vi "Find Register Offset.vi"(8 "error in (no error)":errorcluster, 10 "register name":string, 11 "session in":u32) -> (0 "error out":errorcluster, 2 "resource offset":u32, 3 "session out":u32)   [LabVIEW 2020, in "FPGA Register IO.lvlib"]
uses:
  FPGA Register IO.lvlib
  TypeDefs/Register Data Store.ctl
  NiFpga.dll
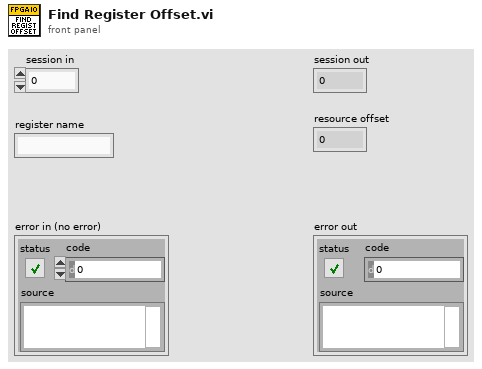
[diagram p1: front panel]
types:
  T1 = typedef "FPGA Register IO.lvlib/Register Data Store.ctl" = cluster{"Register Names":string[], "Register Offset":u32[]}
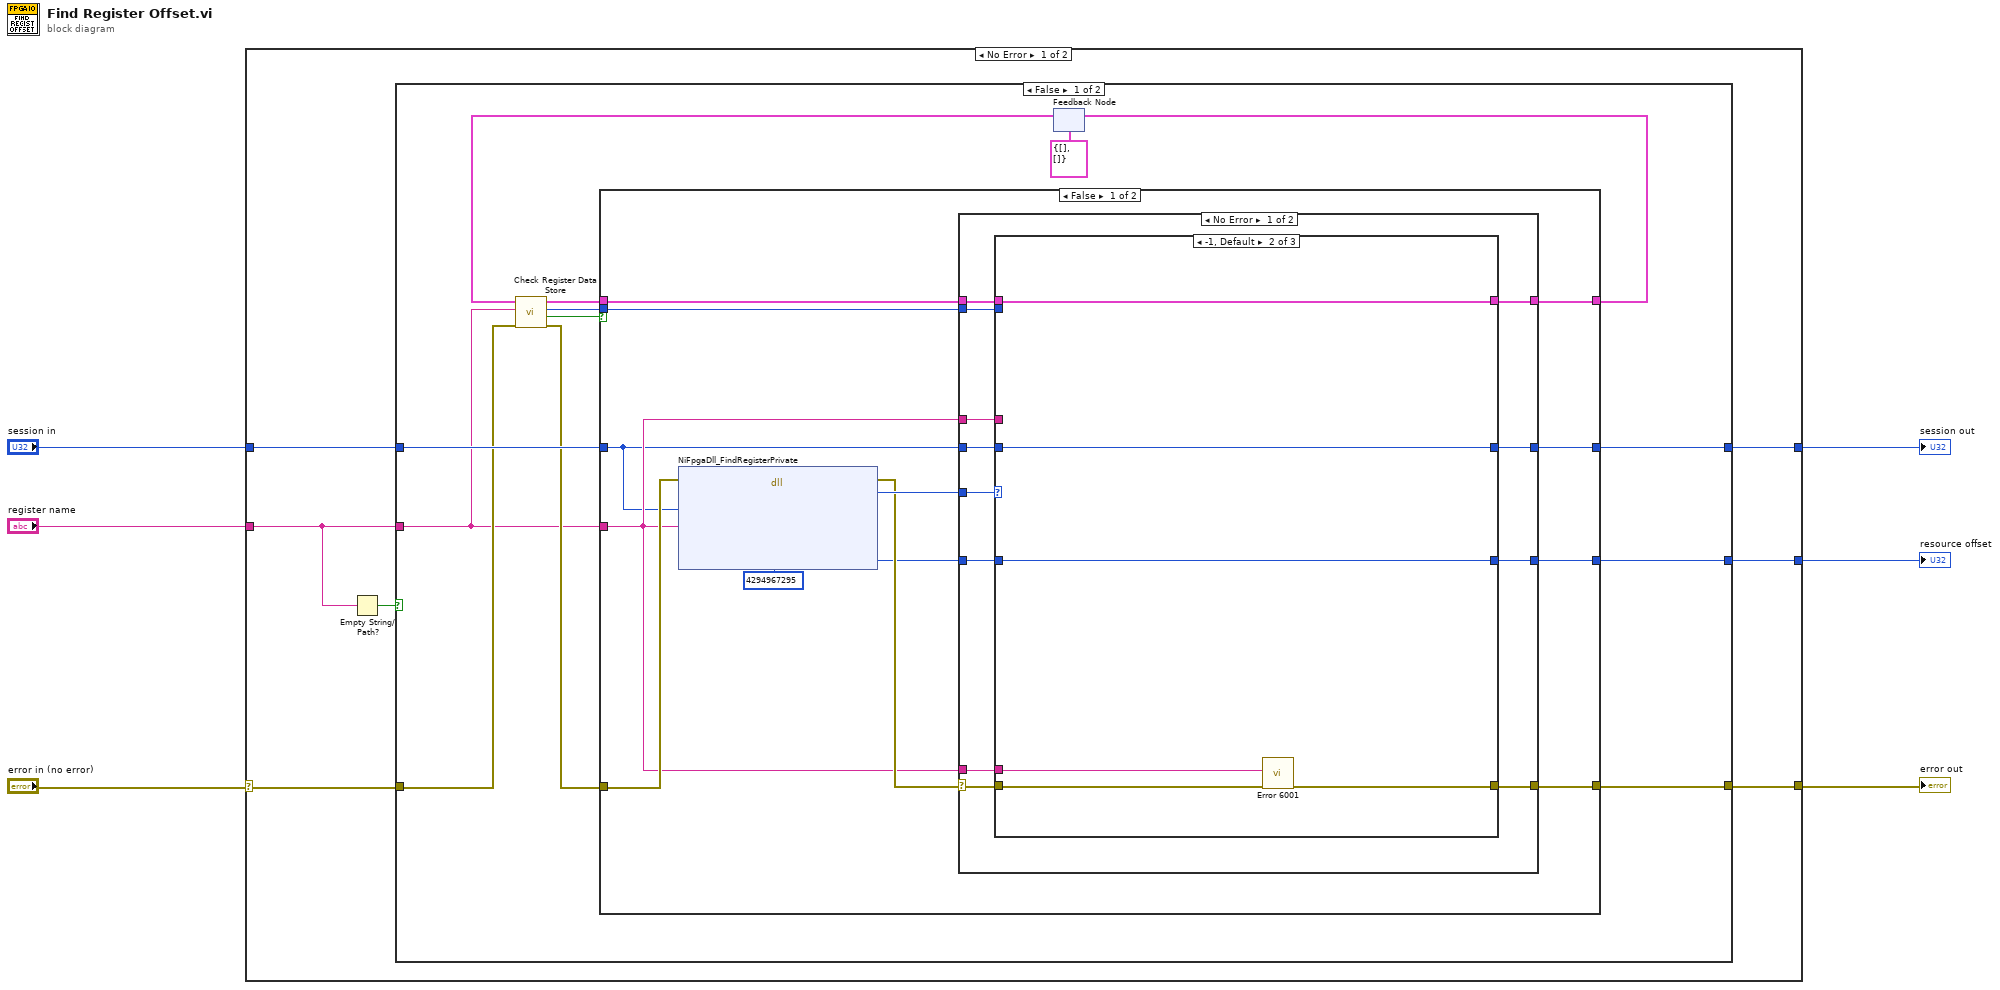
[diagram p0: block diagram]
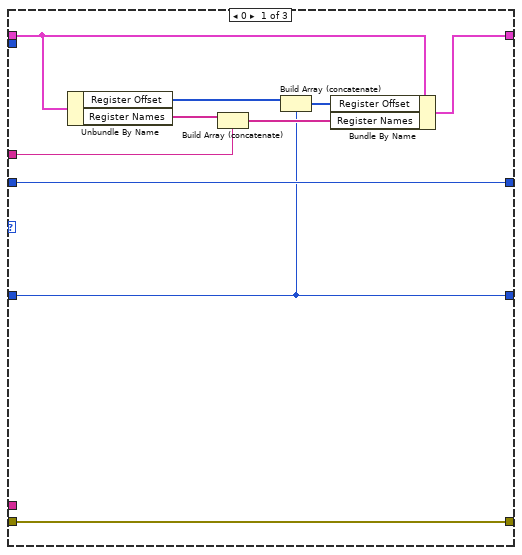
[diagram p2: hidden frame]
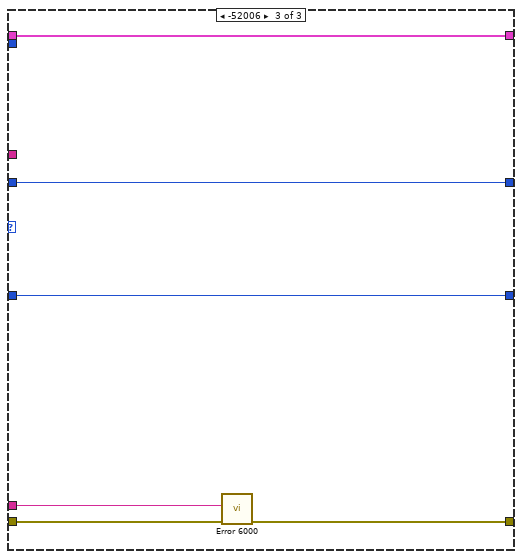
[diagram p3: hidden frame]
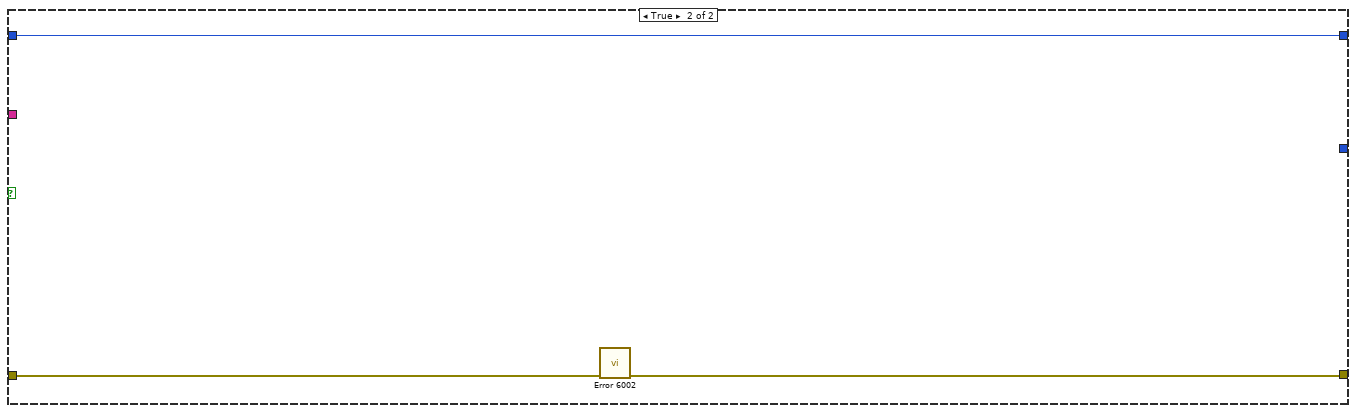
[diagram p6: hidden frame]
diagram:
  n1 = case shown="No Error" "error in (no error)" {
    selector: "error in (no error)" -> [w9 w86]
    tunnel: [w12 w86] -> w3
    tunnel: "register name" -> [w8 _]
    tunnel: "session in" -> [w13 w85]
    tunnel: [w11 w85] -> w4
    tunnel: [w10 _] -> w2
    frame No Error {
      n2 = Empty String/Path?(string/path=w8) -> (empty?=w7:bool)
      n3 = case shown="False" w7 {
        tunnel: w13 -> [w26 w82]
        tunnel: [w25 w83] -> w12
        tunnel: [w24 w82] -> w11
        tunnel: [w23 _] -> w10
        tunnel: w9 -> [w17 w84]
        tunnel: w8 -> [w14 _]
        frame False {
          n4 = feedback #1(T1 {"Register Names"=[], "Register Offset"=[]}) -> (w21:T1)
          n5 = call "Check Register Data Store.vi"("error in (no error)"=w17, "register name"=w14, "register data store in"=w21) -> ("error IO"=w16:errorcluster, "Found"=w15:bool, "register offset"=w19:u32, "register data store out"=w20:T1)  [unwired: 5 in]
          n6 = case shown="False" w15 {
            tunnel: w16 -> [w38 w80]
            tunnel: w26 -> [w29 w81]
            tunnel: [w27 w78] -> w23
            tunnel: [w36 w80] -> w25
            tunnel: [w28 w81] -> w24
            tunnel: w14 -> [w32 _]
            tunnel: w20 -> [w34 w79]
            tunnel: w19 -> [w33 w78]
            tunnel: [w30 w79] -> w18
            frame False {
              n7 = dll-call lib="NiFpga.*" fn="NiFpgaDll_FindRegisterPrivate"(error in=w38, "session"=w29, "registerName"=w32, "expectedResourceType"=u32 4294967295) -> (error out=w35:errorcluster, "status"=w37:i32, "resourceOffset"=w31:u32)  [unwired: 6 in, 1 out]
              n8 = case shown="No Error" w35 {
                selector: w35 -> [w48 w77]
                tunnel: w37 -> [w51 _]
                tunnel: [w50 w77] -> w36
                tunnel: w32 -> [w49 _]
                tunnel: w34 -> [w47 w74]
                tunnel: w33 -> [w46 _]
                tunnel: w32 -> [w45 _]
                tunnel: w31 -> [w44 w75]
                tunnel: [w43 w74] -> w30
                tunnel: w29 -> [w42 w76]
                tunnel: [w41 w76] -> w28
                tunnel: [w40 w75] -> w27
                frame No Error {
                  n9 = case shown="-1, Default" w51 {
                    tunnel: [w61 w62 w73] -> w50
                    tunnel: w49 -> [_ w63 w68]
                    tunnel: w48 -> [w61 w64 w72]
                    tunnel: w47 -> [w55 w67 w70]
                    tunnel: w46 -> [_ _ _]
                    tunnel: w45 -> [w58 _ _]
                    tunnel: w44 -> [w52 w65 w69]
                    tunnel: [w54 w67 w70] -> w43
                    tunnel: w42 -> [w53 w66 w71]
                    tunnel: [w53 w66 w71] -> w41
                    tunnel: [w52 w65 w69] -> w40
                    frame 0 {
                      n10 = Unbundle By Name(w55) -> ("Register Offset"=w60:u32[], "Register Names"=w59:string[])
                      n11 = Build Array (concatenate)(w59, w58) -> (w56:string[])
                      n12 = Build Array (concatenate)(w60, w52) -> (w57:u32[])
                      n13 = Bundle By Name(cluster=w55, "Register Offset"=w57, "Register Names"=w56) -> (w54:T1)
                    }
                    frame -1, Default {
                      n14 = call "Error 6001.vi"("error in (no error)"=w64, "register name"=w63) -> ("error out"=w62:errorcluster)  [unwired: 9 in]
                    }
                    frame -52006 {
                      n15 = call "Error 6000.vi"("error in (no error)"=w72, "register name"=w68) -> ("error out"=w73:errorcluster)  [unwired: 9 in]
                    }
                  }
                }
                frame Error {
                }
              }
            }
            frame True {
            }
          }
          n16 = feedback-in #1(w18) -> ()
        }
        frame True {
          n17 = call "Error 6002.vi"("error in (no error)"=w84) -> ("error out"=w83:errorcluster)  [unwired: 10 in]
        }
      }
    }
    frame Error {
    }
  }
  "session out" <- w4
  "error out" <- w3
  "resource offset" <- w2
